vi "PowerGuardStart.vi"(0 "Device Info":T1={"Serial Number"=-1, "Channel"=0, "Port"=0}, 5 "Over Voltage":dbl=-1.0, 7 "Fan Mode":u32(ring)=3 items=["FAN_MODE_OFF"=1, "FAN_MODE_ON"=2, "FAN_MODE_AUTO"=3], 9 "Enabled":bool caption="Power Enabled", 11 "error in (no error)":errorcluster, 12 "Connection":u16(ring) items=["No Preference", "Remote", "Local"], 13 "Timeout (mSec)":i32=5000) -> (4 "Phidget ID":u64, 6 "Serial Number Return":i32, 10 "Attached?":bool, 15 "error out":errorcluster)   [LabVIEW 2020, in "Phidget Power Guard.lvlib"]
doc: "${PowerGuard:StartHeader}"
uses:
  <instrlib>/Phidgets/Phidget Power Guard/Phidget Power Guard.lvlib
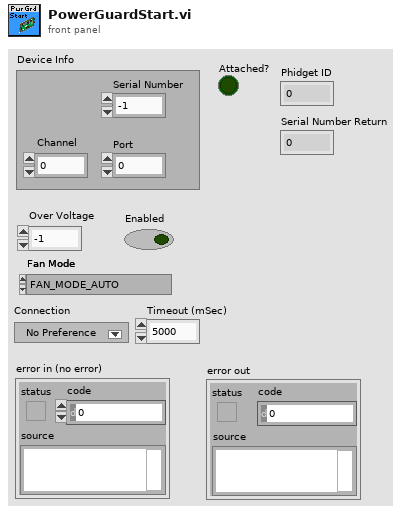
[diagram p1: front panel]
types:
  T1 = cluster{"Serial Number":i32, "Channel":i32, "Port":i32}
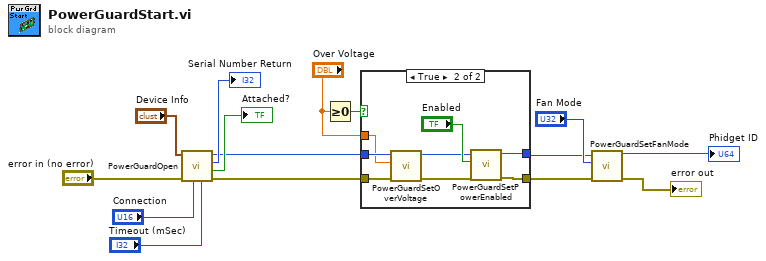
[diagram p0: block diagram]
diagram:
  n1 = call <instrlib>:"PowerGuardOpen.vi"("Timeout (mSec)"="Timeout (mSec)", "Connection"="Connection", "error in"="error in (no error)", "Device Info"="Device Info") -> ("error out"=w6:errorcluster, "Attached?"=→"Attached?":bool, "Serial Number Return"=→"Serial Number Return":i32, "Phidget ID"=w7:u64)  [unwired: 4 in]
  n2 = Greater Or Equal To 0?(x="Over Voltage") -> (x >= 0?=w8:bool)
  n3 = case shown="True" w8 {
    tunnel: w7 -> [w17 w24]
    tunnel: w6 -> [w16 w25]
    tunnel: "Over Voltage" -> [_ w23]
    tunnel: [w17 w19] -> w4
    tunnel: [w16 w18] -> w3
    frame False {
    }
    frame True {
      n4 = call <instrlib>:"PowerGuardSetOverVoltage.vi"("error in (no error)"=w25, "Over Voltage"=w23, "Device In"=w24) -> ("error out"=w20:errorcluster, "Device Out"=w21:u64)  [unwired: 6 in]
      n5 = call <instrlib>:"PowerGuardSetPowerEnabled.vi"("error in (no error)"=w20, "Enabled"="Enabled", "Device In"=w21) -> ("error out"=w18:errorcluster, "Device Out"=w19:u64)  [unwired: 6 in]
    }
  }
  n6 = call <instrlib>:"PowerGuardSetFanMode.vi"("error in (no error)"=w3, "Fan Mode"="Fan Mode", "Device In"=w4) -> ("error out"=→"error out":errorcluster, "Device Out"=→"Phidget ID":u64)  [unwired: 6 in]
